vi "Streaming.vi"() -> ()   [LabVIEW 2025]
uses:
  <vilib>/Utility/file.llb/Write Delimited Spreadsheet (DBL).vi
panel:
  out "Waveform Chart":dbl[][](graph)
  in  "stop 2":bool
  out "Error":errorcluster
  out "Error String":string
  out "Connected?":bool
  out "Actual SampleRate (Hz)":dbl format="%.3f"
  out "NumAddresses":i32
  in  "STREAM_RESOLUTION_INDEX":i32
  in  "STREAM_SETTLING_US":i32
  in  "AIN_ALL_RANGE":dbl=10.0 format="%.3f"
  out "ScansPerRead":i32
  out "ConnectionType Out":i32
  out "DeviceType Out":i32
  out "# of iterations":i32
  out "Data":dbl[][](array[numeric]) format="%.3f"
  out "LJMScanBacklog":i32
  out "DeviceScanBacklog":i32
  in  "Seconds on Graph":dbl=1.0 format="%.2f"
  in  "Scan List":string[](array[string])=["AIN0", "AIN1", "AIN2", "AIN3"]
  in  "Scan Rate (Hz)":dbl=1000.0 format="%.3f"
  # "LabJack"
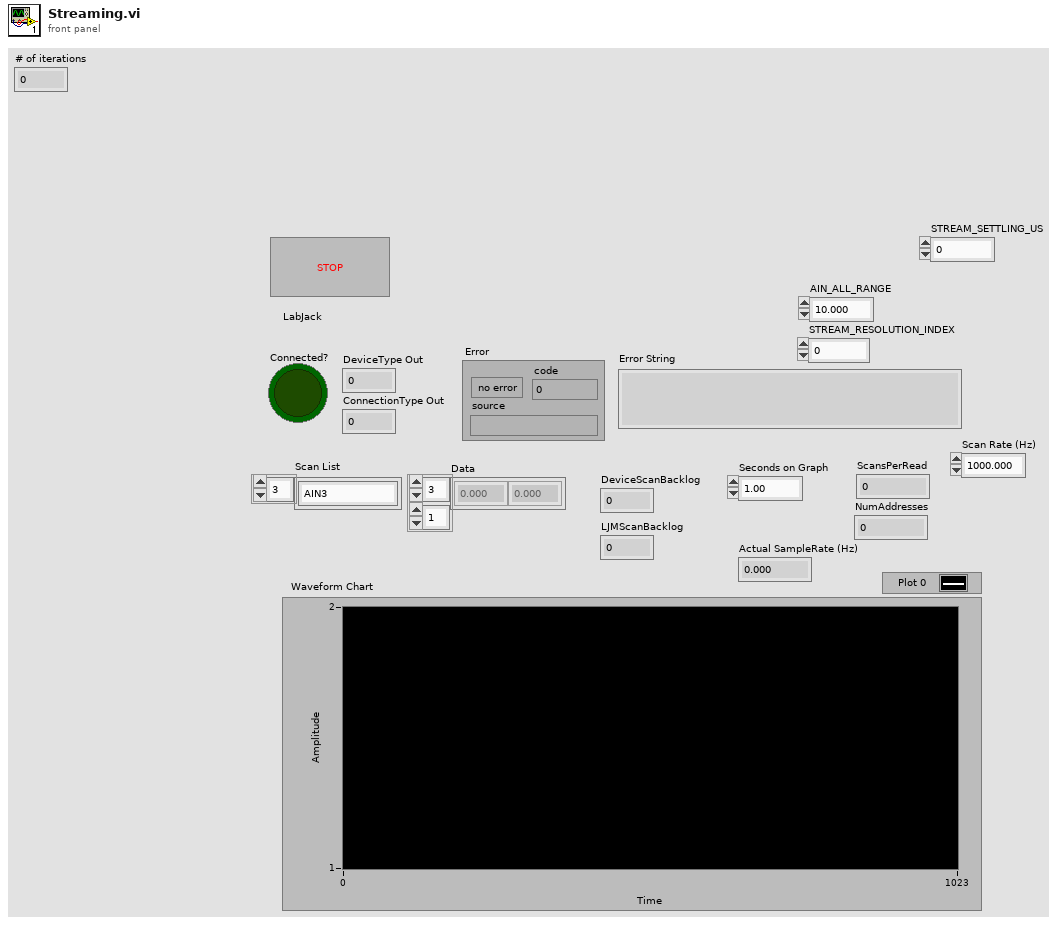
[diagram p1: front panel]
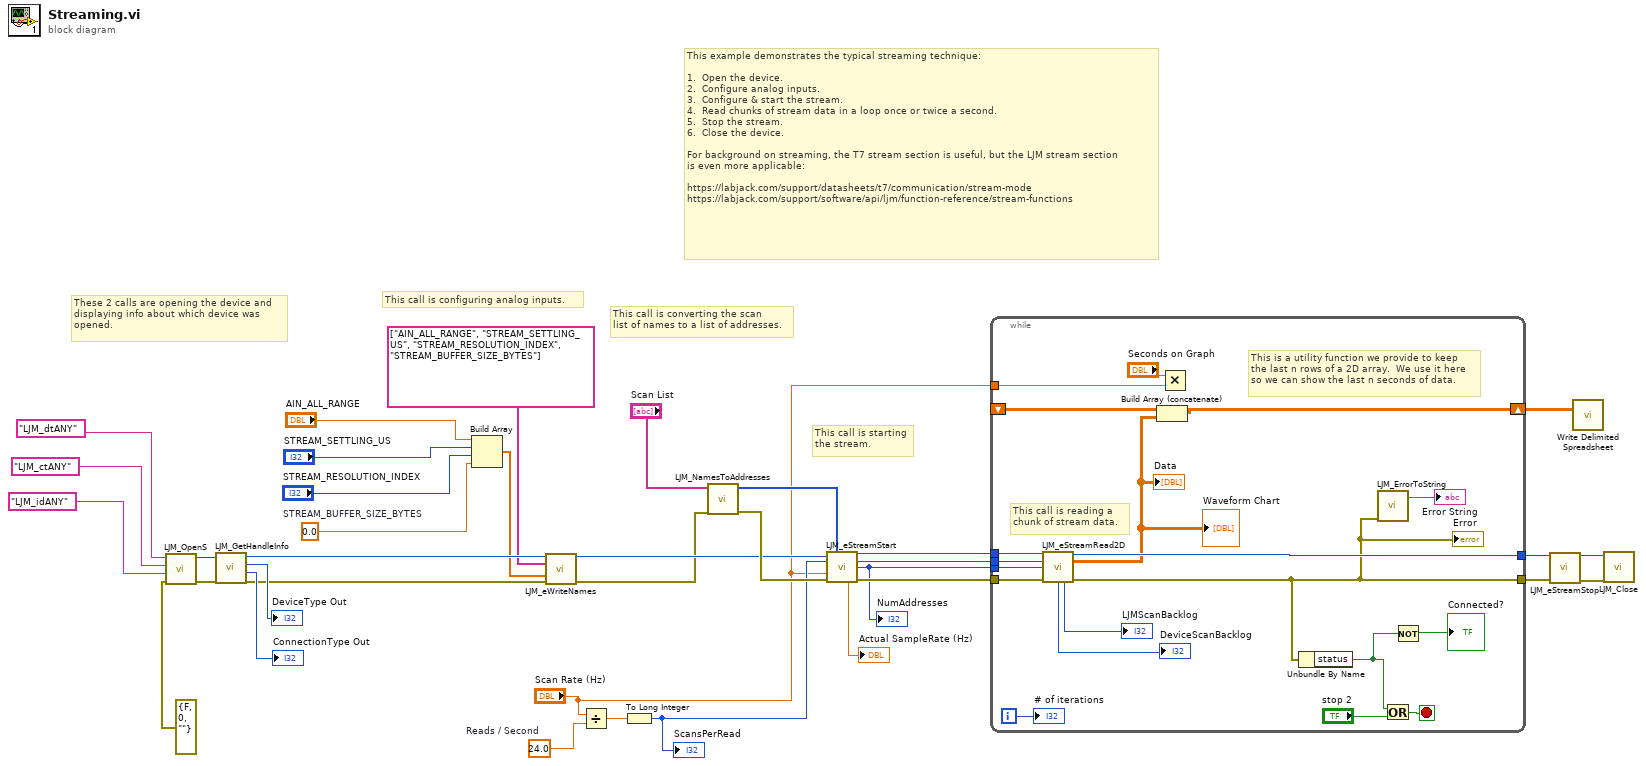
[diagram p0: block diagram]
diagram:
  w7 = 0.0  # STREAM_BUFFER_SIZE_BYTES
  w24 = 24.0  # Reads / Second
  # "This example demonstrates the typical streaming technique:\n\n1.  Open the device.\n2.  Configure analog inputs.\n3.  Configure & start the stream.\n4.  Read chunks of stream data in a loop once or twice a second.\n5.  Stop the stream.\n6.  Close the device.\n\nFor background on streaming, the T7 stream section is useful, but the LJM stream section\nis even more applicable:\n\nhttps://labjack.com/support/datasheets/t7/communication/stream-mode\nhttps://labjack.com/support/software/api/ljm/function-reference/stream-functions"
  # "This call is starting\nthe stream."
  # "This call is converting the scan\nlist of names to a list of addresses."
  # "This call is configuring analog inputs."
  # "These 2 calls are opening the device and\ndisplaying info about which device was\nopened."
  n1 = call <vilib>:"LJM_OpenS.vi"("error in"=errorcluster {"status"=FALSE, "code"=0, "source"=""} ("error in (no error)"), "Identifier"="LJM_idANY", "ConnectionType"="LJM_ctANY", "DeviceType"="LJM_dtANY") -> ("error out"=w29:errorcluster, "Handle"=w28:i32)  [unwired: 6 in]
  n2 = call <vilib>:"LJM_GetHandleInfo.vi"("error in"=w29, "Handle In"=w28) -> ("error out"=w21:errorcluster, "ConnectionType"=→"ConnectionType Out":i32, "DeviceType"=→"DeviceType Out":i32, "Handle Out"=w20:i32)  [unwired: 2 in, 4 out]
  n3 = Build Array("AIN_ALL_RANGE", "STREAM_SETTLING_US", "STREAM_RESOLUTION_INDEX", w7) -> (w15:dbl[])
  n4 = call <vilib>:"LJM_eWriteNames.vi"("Handle In"=w20, "aNames"=string[] ["AIN_ALL_RANGE", "STREAM_SETTLING_US", "STREAM_RESOLUTION_INDEX", "STREAM_BUFFER_SIZE_BYTES"], "aValuesIn"=w15, "error in"=w21) -> ("Handle Out"=w19:i32, "error out"=w18:errorcluster)  [unwired: 9 in, 1 out]
  n5 = Divide(x="Scan Rate (Hz)", y=w24) -> (x/y=w23:dbl)
  n6 = To Long Integer(number=w23) -> (32bit integer=w22:i32)
  "ScansPerRead" <- w22
  n7 = call <vilib>:"LJM_NamesToAddresses.vi"("error in"=w18, "aNames"="Scan List") -> ("error out"=w25:errorcluster, "aAddresses"=w12:i32[])  [unwired: 7 in, 1 out]
  n8 = call <vilib>:"LJM_eStreamStart.vi"("Handle In"=w19, "aScanList"=w12, "ScansPerRead"=w22, "ScanRate"="Scan Rate (Hz)", "error in"=w25) -> ("Handle Out"=w34:i32, "ScansPerRead Out"=w8:i32, "NumReadAddresses"=w10:i32, "Actual SampleRate"=→"Actual SampleRate (Hz)":dbl, "error out"=w35:errorcluster)  [unwired: 5 in, 1 out]
  "NumAddresses" <- w10
  n9 = while {
    tunnel: [w50] -> w32
    tunnel: w34 -> [w51]
    tunnel: w10 -> [w47]
    tunnel: w8 -> [w46]
    shift-right: [w37] -> w1
    shift-left: _ -> [w44]
    tunnel: "Scan Rate (Hz)" -> [w43]
    tunnel: w35 -> [w52]
    tunnel: [w39] -> w33
    i -> [w53]
    stop <- w54 stop-if-true
    # "This call is reading a\nchunk of stream data."
    # "This is a utility function we provide to keep\nthe last n rows of a 2D array.  We use it here\nso we can show the last n seconds of data."
    n10 = call <vilib>:"LJM_eStreamRead2D.vi"("Handle In"=w51, "ScansPerRead"=w46, "NumAddresses"=w47, "error in"=w52) -> ("Handle Out"=w50:i32, "aData Out"=w36:dbl[][], "DeviceScanBacklog"=→"DeviceScanBacklog":i32, "LJMScanBacklog"=→"LJMScanBacklog":i32, "error out"=w39:errorcluster)  [unwired: 7 in]
    "Data" <- w36
    "Error" <- w39
    "Waveform Chart" <- w36
    n11 = Build Array (concatenate)(w44, w36) -> (w37:dbl[][])
    n12 = Multiply(x="Seconds on Graph", y=w43) -> ()  [unwired: 1 out]
    n13 = Unbundle By Name(w39) -> ("status"=w42:bool)
    n14 = call <vilib>:"LJM_ErrorToString.vi"("error in"=w39) -> ("String"=→"Error String":string)  [unwired: 10 in]
    n15 = Or(x=w42, y="stop 2") -> (x .or. y?=w54:bool)
    n16 = Not(x=w42) -> (.not. x?=→"Connected?":bool)
    "# of iterations" <- w53
  }
  n17 = call <vilib>:"LJM_eStreamStop.vi"("Handle In"=w32, "error in"=w33) -> ("Handle Out"=w30:i32, "error out"=w31:errorcluster)  [unwired: 12 in]
  n18 = call-poly <vilib>:"Write Delimited Spreadsheet.vi"("2D data"=w1) -> ()  [unwired: 13 in, 2 out]
  n19 = call <vilib>:"LJM_Close.vi"("error in"=w31, "Handle"=w30) -> ()  [unwired: 9 in, 1 out]
